vi "Mono Shutter.vi"(8 "error in (no error)":errorcluster, 11 "Mono In":refnum<class "Monochromator.lvclass">) -> (0 "error out":errorcluster, 2 "shutterPosition":i32, 3 "shutterIndex":i32)   [LabVIEW 2023, in "Examples.lvlib"]
doc: "This example shows how to get and set the shutter position of the mono.\n\nNote: this example will return an error if no internal shutter is available."
uses:
  Examples.lvlib
  Classes/Mono/Monochromator.lvclass
panel:
  # "Connector Pane"
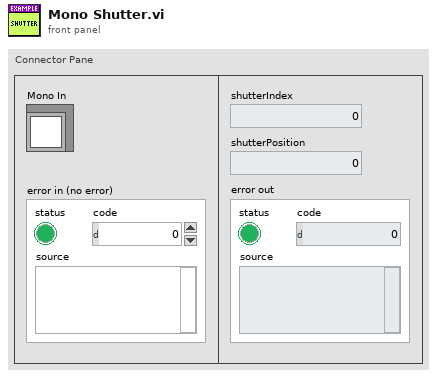
[diagram p1: front panel]
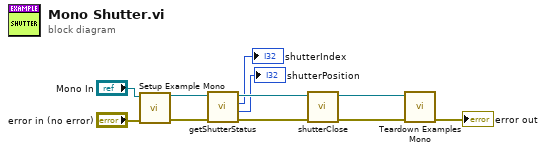
[diagram p0: block diagram]
diagram:
  n1 = call "Setup Example Mono.vi"("error in (no error)"="error in (no error)", "Mono In"="Mono In") -> ("error out"=w8:errorcluster, "Mono Out"=w6:refnum<class "Monochromator.lvclass">)  [unwired: 6 in, 2 out]
  n2 = call "getShutterStatus.vi"("error in (no error)"=w8, "Monochromator in"=w6) -> ("error out"=w7:errorcluster, "shutterPosition"=→"shutterPosition":i32, "shutterIndex"=→"shutterIndex":i32, "Monochromator out"=w5:refnum<class "Monochromator.lvclass">)  [unwired: 6 in]
  n3 = call "shutterClose.vi"("error in (no error)"=w7, "Monochromator in"=w5) -> ("error out"=w2:errorcluster, "Monochromator out"=w1:refnum<class "Monochromator.lvclass">)  [unwired: 6 in, 2 out]
  n4 = call "Teardown Examples Mono.vi"("error in (no error)"=w2, "Monochromator in"=w1) -> ("error out"=→"error out":errorcluster)  [unwired: 9 in]
